vi "Mark Selected Channel in Graph and Multicolumn Listbox.vi"(7 "selected channel":i32, 8 "error in":errorcluster, 10 "Value Table":refnum<vi>, 11 "WaveformGraph":refnum<vi>) -> (0 "error out":errorcluster)   [LabVIEW 2020, in "TdmsFileViewer.lvlib"]
uses:
  TdmsFileViewer.lvlib
  <vilib>/Utility/miscctls.llb/LVRowAndColumnTypeDef.ctl
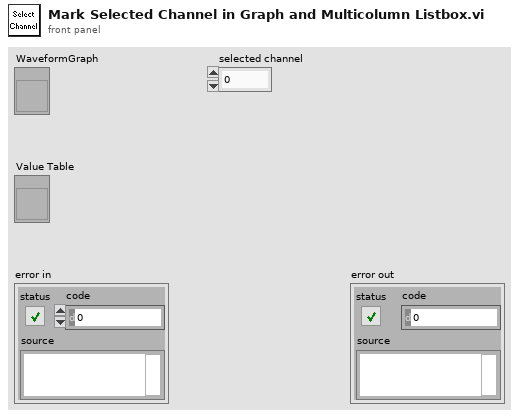
[diagram p1: front panel]
types:
  T1 = typedef "LVRowAndColumnTypeDef.ctl" = cluster{"Row":i32, "Column":i32}
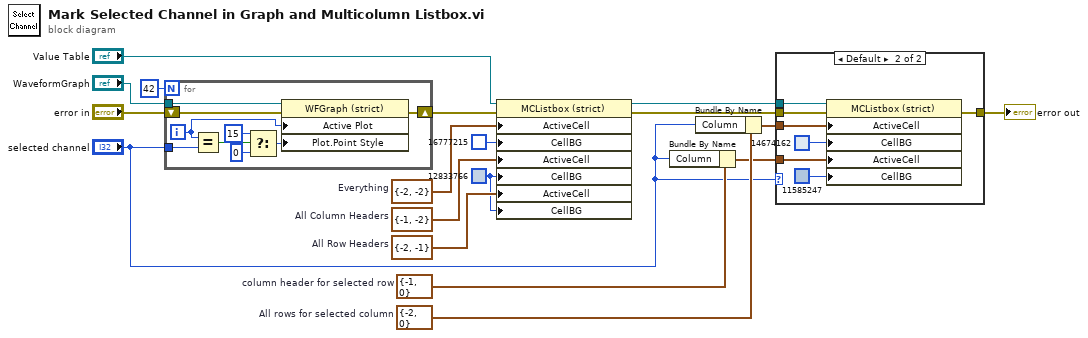
[diagram p0: block diagram]
diagram:
  w4 = T1 {"Row"=-1, "Column"=0}  # column header for selected row
  w7 = T1 {"Row"=-2, "Column"=-1}  # All Row Headers
  w13 = T1 {"Row"=-2, "Column"=0}  # All rows for selected column
  w10 = T1 {"Row"=-1, "Column"=-2}  # All Column Headers
  w12 = T1 {"Row"=-2, "Column"=-2}  # Everything
  w6 = u32 12833766
  n1 = for {
    N: 42 -> [_]
    tunnel: "WaveformGraph" -> [w25]
    tunnel: "selected channel" -> [w20]
    shift-right: [w27] -> w17
    shift-left: "error in" -> [w26]
    i -> [w19]
    n2 = Equal?(x=w19, y=w20) -> (x = y?=w24:bool)
    n3 = Select(t=u8 15 ("Plot.Point Style"), s=w24, f=u8 0) -> (s? t:f=w21:u8)
    n4 = property class="WFGraph (strict)"(reference=w25, error in=w26, "Active Plot"=w19, "Plot.Point Style"=w21) -> (error out=w27:errorcluster)  [unwired: 1 out]
  }
  n5 = property on="Property Node" class="MCListbox (strict)"(reference="Value Table", error in=w17, "ActiveCell"=w12, "CellBG"=u32 16777215, "ActiveCell"=w10, "CellBG"=w6, "ActiveCell"=w7, "CellBG"=w6) -> (reference out=w5:refnum<vi>, error out=w16:errorcluster)
  n6 = Bundle By Name(cluster=w4, "Column"="selected channel") -> (w1:T1)
  n7 = Bundle By Name(cluster=w13, "Column"="selected channel") -> (w2:T1)
  n8 = case shown="Default" "selected channel" {
    tunnel: w5 -> [_ w33]
    tunnel: w16 -> [w28 w35]
    tunnel: [w28 w34] -> w15
    tunnel: w2 -> [_ w32]
    tunnel: w1 -> [_ w31]
    frame ..-1 {
      # "row header selected\ndeselect all channels"
    }
    frame Default {
      n9 = property on="Property Node" class="MCListbox (strict)"(reference=w33, error in=w35, "ActiveCell"=w32, "CellBG"=u32 14674162, "ActiveCell"=w31, "CellBG"=u32 11585247) -> (error out=w34:errorcluster)  [unwired: 1 out]
    }
  }
  "error out" <- w15
